vi "Elevator Encoder Activate.vi"() -> (3 "Distance":dbl)   [LabVIEW 2012]
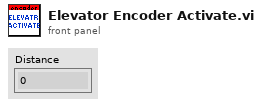
[diagram p1: front panel]
types:
  T1 = typedef "WPI_DigitalInputDevRef.ctl" = cluster{"DevStatus":errorcluster, "DIO Channel":T2, "Digital Module":T3}
  T2 = typedef "FPGA_DIOChannel.ctl" = enum8{"DIO 1", "DIO 2", "DIO 3", "DIO 4", "DIO 5", "DIO 6", "DIO 7", "DIO 8", "DIO 9", "DIO 10", "DIO 11", "DIO 12", "DIO 13", "DIO 14", "Invalid"}
  T3 = typedef "FPGA_TypedefDigitalModule.ctl" = enum16{"Digital Module 1", "Digital Module 2"}
  T4 = typedef "WPI_EncoderDevRef.ctl" = cluster{"DevStatus":errorcluster, "EncoderIndex":T5, "CounterIndex":T6, "DistancePerCount":dbl, "Decoding Type":T7}
  T5 = typedef "FPGA_EncoderIdx.ctl" = enum8{"Enc 0", "Enc 1", "Enc 2", "Enc 3", "Invalid"}
  T6 = typedef "FPGA_CounterCtrSystemIndex.ctl" = enum8{"Ctr 0", "Ctr 1", "Ctr 2", "Ctr 3", "Ctr 4", "Ctr 5", "Ctr 6", "Ctr 7", "Invalid"}
  T7 = typedef "WPI_EncoderType.ctl" = enum16{"1x", "2x", "4x"}
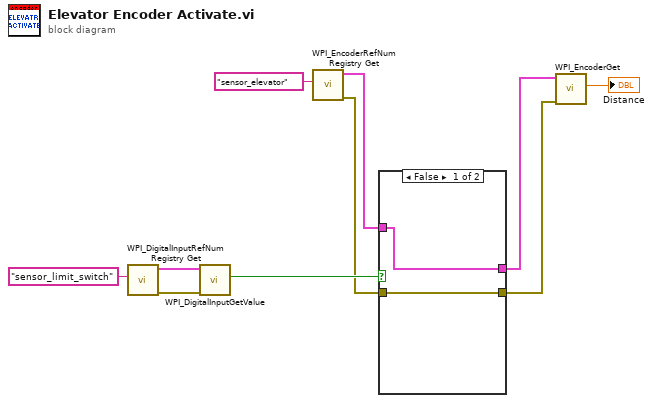
[diagram p0: block diagram]
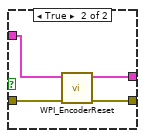
[diagram p2: hidden frame]
diagram:
  n1 = call <vilib>:"WPI_DigitalInputRefNum Registry Get.vi"("refnum name"="sensor_limit_switch") -> ("error out"=w7:errorcluster, "DigitalInputDevRef"=w8:T1)  [unwired: 9 in]
  n2 = call <vilib>:"WPI_DigitalInputGetValue.vi"("error in (no error)"=w7, "DigitalInputDevRef"=w8) -> ("Value"=w5:bool)  [unwired: 7 in, 2 out]
  n3 = call <vilib>:"WPI_EncoderRefNum Registry Get.vi"("refnum name"="sensor_elevator") -> ("error out"=w3:errorcluster, "EncoderDevRef"=w4:T4)  [unwired: 9 in]
  n4 = case shown="False" w5 {
    tunnel: w4 -> [w12 w16]
    tunnel: w3 -> [w11 w15]
    tunnel: [w12 w14] -> w2
    tunnel: [w11 w13] -> w1
    frame False {
    }
    frame True {
      n5 = call <vilib>:"WPI_EncoderReset.vi"("error in (no error)"=w15, "EncoderDevRef"=w16) -> ("error out"=w13:errorcluster, "EncoderDevRef"=w14:T4)  [unwired: 8 in]
    }
  }
  n6 = call <vilib>:"WPI_EncoderGet.vi"("error in (no error)"=w1, "EncoderDevRef"=w2) -> ("Distance"=→"Distance":dbl)  [unwired: 4 in, 5 out]
